vi "SUB-BLE Rx data save.vi"(5 "BLE RxD":u8[](array[numeric])) -> ()   [LabVIEW 2015]
doc: "Use this template to create an application that executes repeatedly until you click the Stop button. This template polls the state of the Stop button and does not use events. Use the Top-Level Application template (not available in the Base package) to create a single-loop application with event handling."
uses:
  Global 1.vi
panel:
  out "BLE Packet (buf)":u8[](array[numeric])
  out "BLE Packet (data)":u8[](array[numeric])
  out "BLE Packet":bool=TRUE
  # "BLE 수신 데이터 처리: 수신 버퍼에 저장."
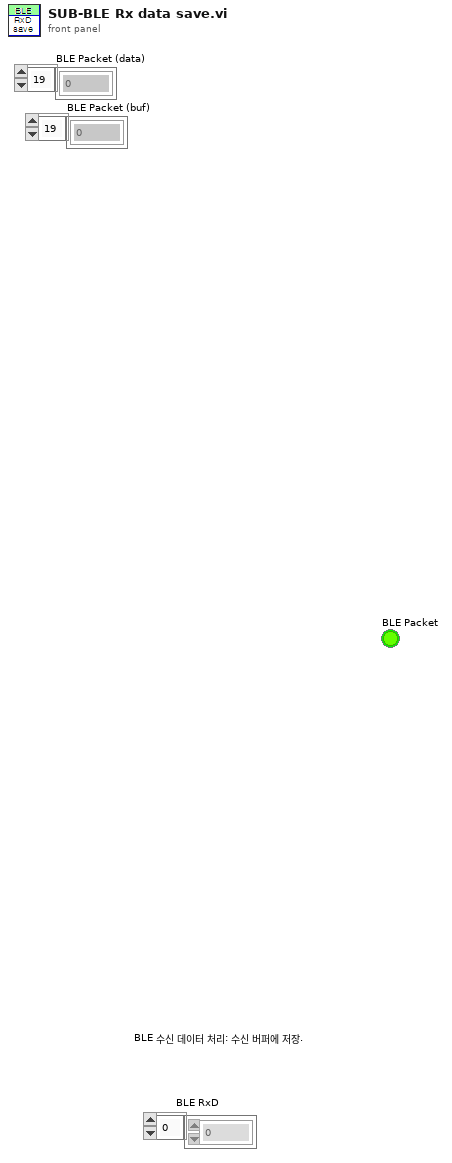
[diagram p1: front panel]
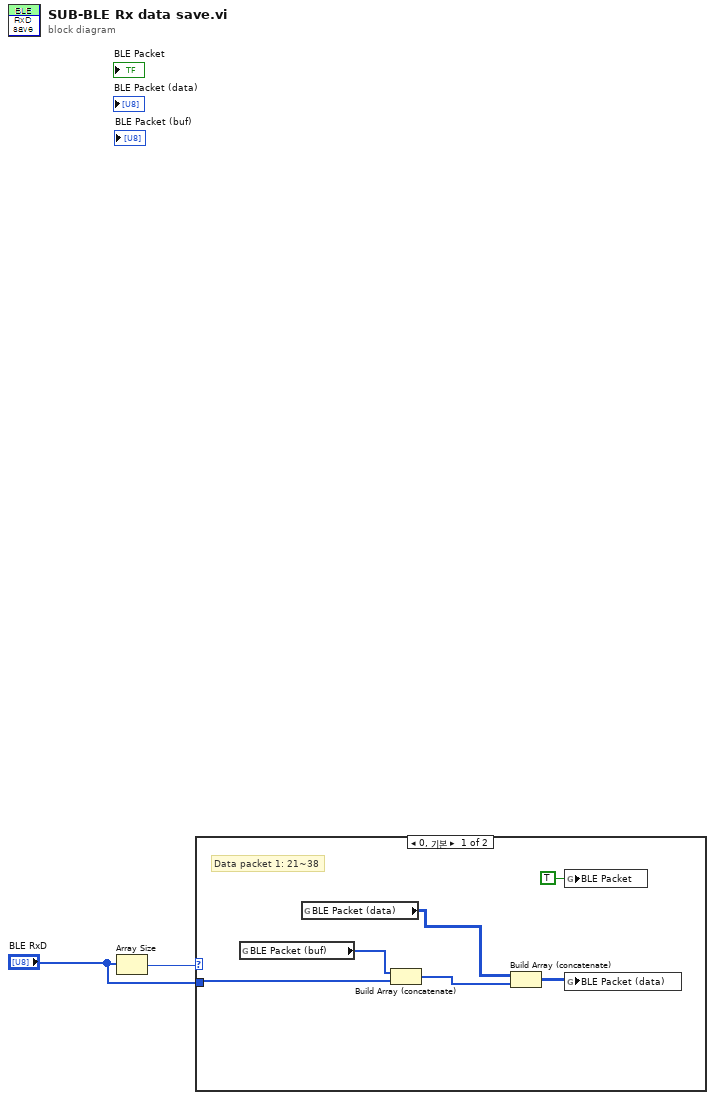
[diagram p0: block diagram]
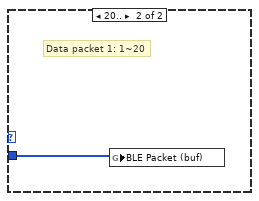
[diagram p2: hidden frame]
diagram:
  n1 = Array Size(array="BLE RxD") -> (size(s)=w2:i32)
  n2 = case shown="0, 기본" w2 {
    tunnel: "BLE RxD" -> [w8 w9]
    frame 0, Default {
      # "Data packet 1: 21~38"
      n3 = global read "Global 1.vi" "BLE Packet (buf)"() -> (w6:u8[])
      n4 = global read "Global 1.vi" "BLE Packet (data)"() -> (w5:u8[][])
      n5 = Build Array (concatenate)(w6, w8) -> (w3:u8[])
      n6 = Build Array (concatenate)(w5, w3) -> (w4:u8[][])
      n7 = global write "Global 1.vi" "BLE Packet"(TRUE ("BLE Packet")) -> ()
      n8 = global write "Global 1.vi" "BLE Packet (data)"(w4) -> ()
    }
    frame 20.. {
      # "Data packet 1: 1~20"
      n9 = global write "Global 1.vi" "BLE Packet (buf)"(w9) -> ()
    }
  }
